vi "final.vi"() -> ()   [LabVIEW 2014]
panel:
  out "Array":i32[][](array[numeric])
  in  "Numeric 2":i32=7
  in  "Numeric":i32
  in  "G 2":dbl[][](array[numeric])
  in  "messages 2":i16[][](array[numeric])
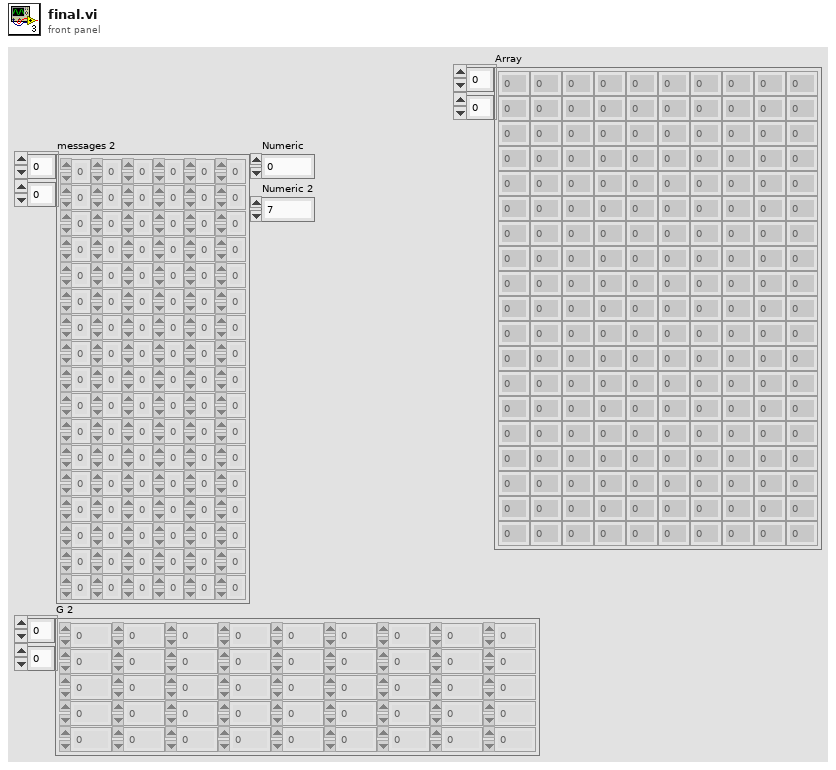
[diagram p1: front panel]
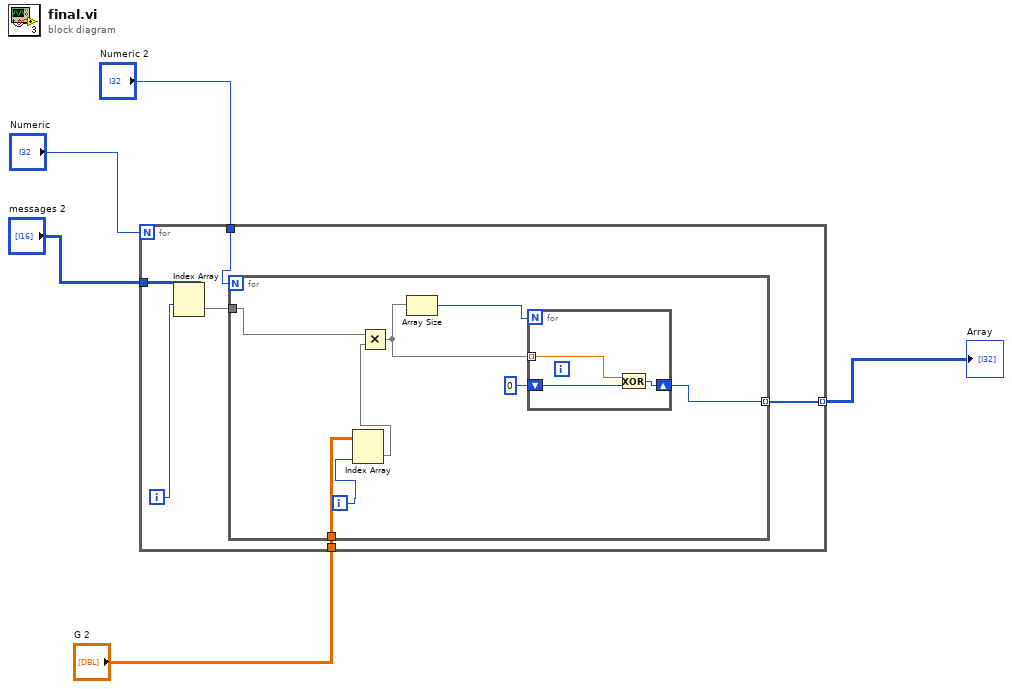
[diagram p0: block diagram]
diagram:
  n1 = for {
    N: "Numeric" -> [_]
    tunnel: "messages 2" -> [w11]
    tunnel: "G 2" -> [w10]
    tunnel: "Numeric 2" -> [w8]
    tunnel: [w7] -> w1 mode=indexing
    i -> [w6]
    n2 = Index Array(array=w11, index (row)=w6) -> (element=w9:i16[])  [unwired: 1 in]
    n3 = for {
      N: w8 -> [_]
      tunnel: w10 -> [w19]
      tunnel: w9 -> [w17]
      tunnel: [w12] -> w7 mode=indexing
      i -> [w13]
      n4 = Index Array(array=w19, index (col)=w13) -> (element=w16:dbl[])  [unwired: 1 in]
      n5 = Multiply(x=w17, y=w16) -> (x*y=w14:dbl[])
      n6 = Array Size(array=w14) -> (size(s)=w15:i32)
      n7 = for {
        N: w15 -> [_]
        tunnel: w14 -> [w20] mode=indexing
        shift-right: [w21] -> w12
        shift-left: 0 -> [w22]
        n8 = Exclusive Or(1:w22, 2:w20) -> (0:w21:i32)
      }
    }
  }
  "Array" <- w1
